vi "Receiver.vi"() -> ()   [LabVIEW 2020]
uses:
  <instrlib>/niUSRP/niUSRP Fetch Rx Data (2D CDB).vi
panel:
  out "Waveform Graph":dbl[][](graph)
  in  "Stop Button":bool
  in  "active antenna":string
  in  "gain":dbl format="%#_6f"
  in  "carrier frequency":dbl=100000.0 format="%#_6p"
  in  "IQ rate":dbl=100000.0 format="%#_6p"
  in  "device names":refnum<k15>
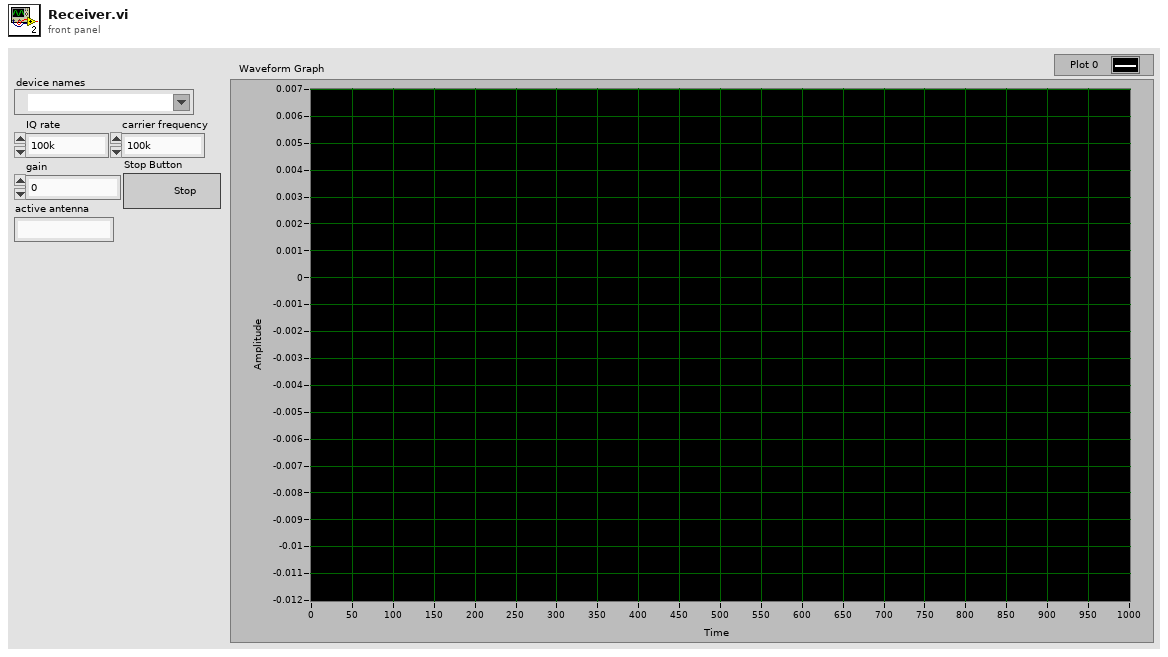
[diagram p1: front panel]
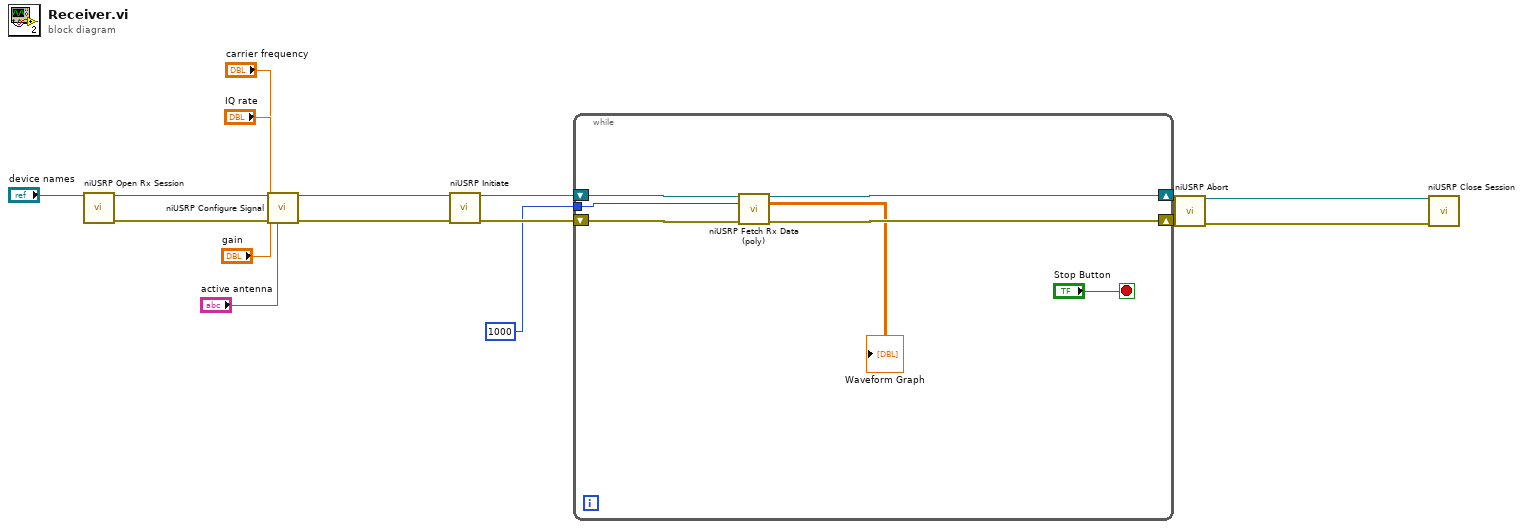
[diagram p0: block diagram]
diagram:
  n1 = call <instrlib>:"niUSRP Open Rx Session.vi"("device names"="device names") -> ("session handle out"=w16:refnum<k15>, "error out"=w15:errorcluster)  [unwired: 13 in]
  n2 = call <instrlib>:"niUSRP Configure Signal.vi"("session handle"=w16, "IQ rate"="IQ rate", "carrier frequency"="carrier frequency", "gain"="gain", "error in (no error)"=w15, "active antenna"="active antenna") -> ("session handle out"=w14:refnum<k15>, "error out"=w13:errorcluster)  [unwired: 5 in, 3 out]
  n3 = call <instrlib>:"niUSRP Initiate.vi"("session handle"=w14, "error in (no error)"=w13) -> ("session handle out"=w12:refnum<k15>, "error out"=w11:errorcluster)  [unwired: 12 in]
  n4 = while {
    shift-right: [w21] -> w10
    shift-left: w12 -> [w23]
    shift-right: [w20] -> w9
    shift-left: w11 -> [w22]
    tunnel: i64 1000 ("number of samples") -> [w18]
    stop <- "Stop Button" stop-if-true
    n5 = call-poly <instrlib>:"niUSRP Fetch Rx Data (poly).vi"("session handle"=w23, "number of samples"=w18, "error in (no error)"=w22) -> ("session handle out"=w21:refnum<k15>, "data"=→"Waveform Graph":cdb[][], "error out"=w20:errorcluster)  [unwired: 9 in, 1 out]
  }
  n6 = call <instrlib>:"niUSRP Abort.vi"("session handle"=w10, "error in (no error)"=w9) -> ("session handle out"=w8:refnum<k15>, "error out"=w7:errorcluster)  [unwired: 12 in]
  n7 = call <instrlib>:"niUSRP Close Session.vi"("session handle"=w8, "error in (no error)"=w7) -> ()  [unwired: 13 in, 1 out]
